vi "VsEP-Set Level.vi"(0 "Runtime":T1, 11 "error in (no error)":errorcluster) -> (4 "Runtime out":T1, 13 "atten":dbl, 14 "Level":dbl, 15 "error out":errorcluster)   [LabVIEW 2020]
uses:
  Typedefs/VsEP-Runtime Data.ctl
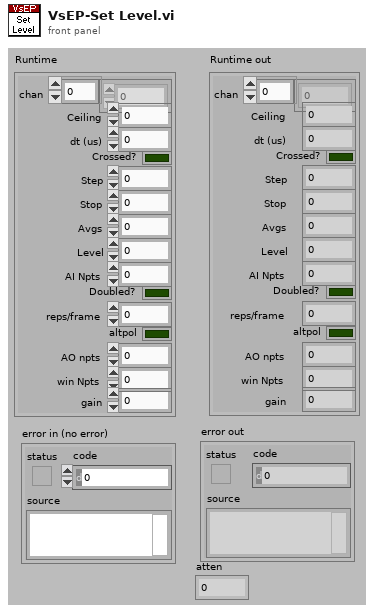
[diagram p1: front panel]
types:
  T1 = typedef "VsEP-Runtime Data.ctl" = cluster{"chan":i32[], "Ceiling":dbl, "dt (us)":dbl, "Crossed?":bool, "Step":dbl, "Stop":i32, "Avgs":i32, "Level":dbl, "AI Npts":i32, "Doubled?":bool, "reps/frame":i32, "altpol":bool, "AO npts":i32, "win Npts":i32, "gain":dbl}
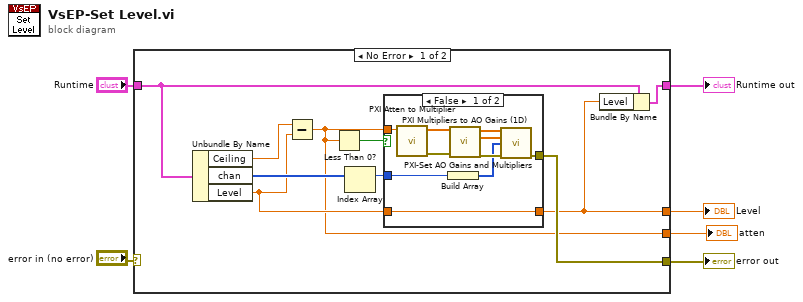
[diagram p0: block diagram]
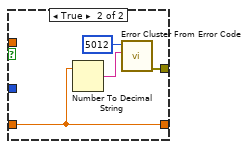
[diagram p2: hidden frame]
diagram:
  n1 = case shown="No Error" "error in (no error)" {
    selector: "error in (no error)" -> [_ w31]
    tunnel: "Runtime" -> [w13 w32]
    tunnel: [w9 w32] -> w4
    tunnel: [w14 w31] -> w3
    tunnel: [w8 _] -> w2
    tunnel: [w7 _] -> w1
    frame No Error {
      n2 = Unbundle By Name(w13) -> ("Ceiling"=w16:dbl, "chan"=w15:i32[], "Level"=w11:dbl)
      n3 = Subtract(x=w16, y=w11) -> (x-y=w7:dbl)
      n4 = Less Than 0?(x=w7) -> (x < 0?=w12:bool)
      n5 = Index Array(array=w15) -> (element=w10:i32)  [unwired: 1 in]
      n6 = case shown="False" w12 {
        tunnel: w7 -> [w26 _]
        tunnel: w10 -> [w20 _]
        tunnel: [w18 w30] -> w14
        tunnel: w11 -> [w17 w27]
        tunnel: [w17 w27] -> w8
        frame False {
          n7 = call "PXI Atten to Multiplier.vi"("Attenuation"=w26) -> ("error out"=w24:errorcluster, "Multiplier setting"=w25:dbl[])  [unwired: 9 in]
          n8 = Build Array(w20) -> (w19:i32[])
          n9 = call "PXI Multipliers to AO Gains (1D).vi"("Multipliers in"=w25, "error in (no error)"=w24) -> ("Multipliers out"=w21:dbl[], "Gains"=w22:dbl[], "error out"=w23:errorcluster)  [unwired: 11 in]
          n10 = call "PXI-Set AO Gains and Multipliers.vi"("Multipliers"=w21, "Gains"=w22, "AO Channels"=w19, "error in (no error)"=w23) -> ("error out"=w18:errorcluster)  [unwired: 11 in]
        }
        frame True {
          n11 = Number To Decimal String(number=w27) -> (decimal integer string=w28:string)  [unwired: 1 in]
          n12 = call <vilib>:"Error Cluster From Error Code.vi"("error message (\"\")"=w28, "error code (0)"=5012) -> ("error out"=w30:errorcluster)  [unwired: 7 in]
        }
      }
      n13 = Bundle By Name(cluster=w13, "Level"=w8) -> (w9:T1)
    }
    frame Error {
    }
  }
  "error out" <- w3
  "Level" <- w2
  "Runtime out" <- w4
  "atten" <- w1
